vi "Set Sender.vi"(10 "Sender":refnum<class "Sender.lvclass">, 11 "Teardown Msg in":refnum<class "Teardown Msg.lvclass">) -> (3 "Teardown Msg out":refnum<class "Teardown Msg.lvclass">)   [LabVIEW 2020, in "jettl.lvlib" / "Teardown Msg.lvlib" / "Teardown Msg.lvclass"]
uses:
  Teardown Msg.lvclass
  Sender/Sender/Sender.lvclass
  Teardown Msg.lvclass/Teardown Msg.ctl
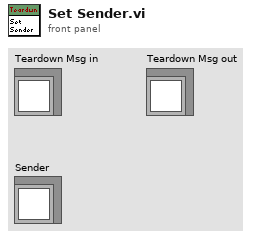
[diagram p1: front panel]
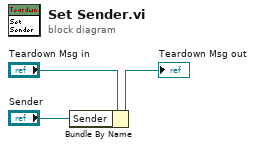
[diagram p0: block diagram]
diagram:
  n1 = Bundle By Name(cluster="Teardown Msg in", "Sender"="Sender") -> (→"Teardown Msg out":refnum<class "Teardown Msg.lvclass">)
